vi "Init Trigger Output.vi"(8 "Error in":errorcluster, 11 "State Variables in":T1={"Stop Notifier"=refnum, "UI References"=[], "DAQmx"={"ECG Input"={"Channel"="", "Task"="", "Max Value"=0.0, "Min Value"=0.0, "Sampling Rate"=0.0, "Batch Size"=10}, "Trigger Output"={"Channel"="", "Task"="", "Pulse Frequency"=0.0, "Delay"=0, "Triggers per Shot"=0}}, "Data Queue"=refnum, "Filter"={"Batch Size"=1000, "Update Cycle"=0, "Filter Buffer"=[]}, "Last Detect Result"=FALSE}) -> (0 "Error out":errorcluster, 3 "State Variables out":T1={"Stop Notifier"=refnum, "UI References"=[], "DAQmx"={"ECG Input"={"Channel"="", "Task"="", "Max Value"=0.0, "Min Value"=0.0, "Sampling Rate"=0.0, "Batch Size"=10}, "Trigger Output"={"Channel"="", "Task"="", "Pulse Frequency"=0.0, "Delay"=0, "Triggers per Shot"=0}}, "Data Queue"=refnum, "Filter"={"Batch Size"=1000, "Update Cycle"=0, "Filter Buffer"=[]}, "Last Detect Result"=FALSE})   [LabVIEW 2014, in "Trigger Output.lvlib"]
uses:
  Trigger Output.lvlib
  Controls/State Variables.ctl
  Controls/DAQmx Variables.ctl
  Controls/Filter Variables.ctl
  <vilib>/DAQmx/create/channels.llb/DAQmx Create Channel (CO-Pulse Generation-Frequency).vi
  <vilib>/DAQmx/configure/timing.llb/DAQmx Timing (Implicit).vi
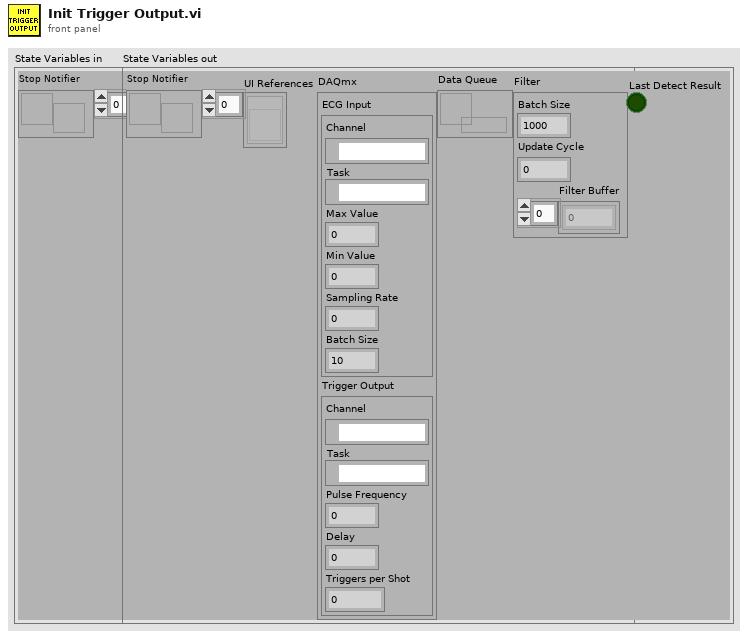
[diagram p1: front panel]
types:
  T1 = typedef "State Variables.ctl" = cluster{"Stop Notifier":refnum<notifier>, "UI References":refnum<vi>[], "DAQmx":T2, "Data Queue":refnum<queue>, "Filter":T3, "Last Detect Result":bool}
  T2 = typedef "DAQmx Variables.ctl" = cluster{"ECG Input":cluster{"Channel":tag, "Task":refnum<k21>, "Max Value":dbl, "Min Value":dbl, "Sampling Rate":dbl, "Batch Size":i32}, "Trigger Output":cluster{"Channel":tag, "Task":refnum<k21>, "Pulse Frequency":dbl, "Delay":u16, "Triggers per Shot":i32}}
  T3 = typedef "Filter Variables.ctl" = cluster{"Batch Size":i32, "Update Cycle":i32, "Filter Buffer":dbl[]}
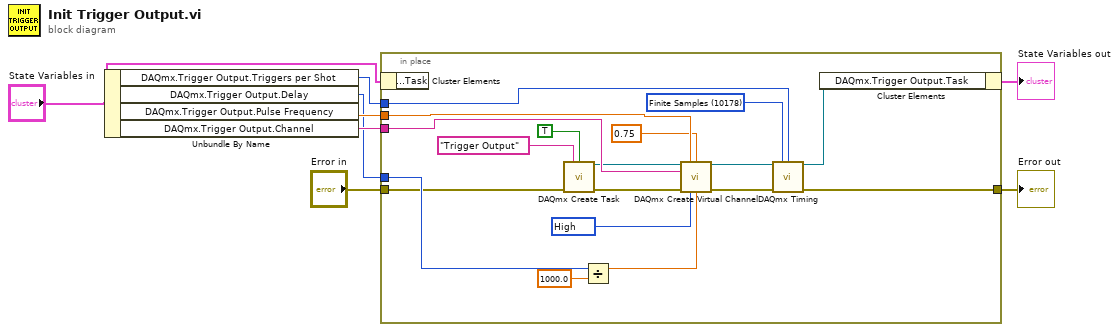
[diagram p0: block diagram]
diagram:
  n1 = Unbundle By Name("State Variables in") -> ("DAQmx.Trigger Output.Triggers per Shot"=w1:i32, "DAQmx.Trigger Output.Delay"=w2:u16, "DAQmx.Trigger Output.Pulse Frequency"=w3:dbl, "DAQmx.Trigger Output.Channel"=w6:tag)
  n2 = in-place {
    in-place-border: w6 -> [w24]
    in-place-border: "Error in" -> [w14]
    in-place-border: [w23] -> w4
    in-place-border: w3 -> [w21]
    in-place-border: w2 -> [w20]
    in-place-border: w1 -> [w17]
    w16 = 10178 items=["Finite Samples"=10178, "Continuous Samples"=10123, "Hardware Timed Single Point"=12522] ("sample mode")
    w19 = 10192 items=["High"=10192, "Low"=10214] ("idle state")
    n3 = in-place-cluster #1("State Variables in") -> ()  [unwired: 1 out]
    n4 = call <vilib>:"DAQmx Create Task.vi"("new task name"="Trigger Output" ("name to assign"), "auto cleanup"=TRUE, "error in"=w14) -> ("task out"=w12:refnum<k21>, "error out"=w13:errorcluster)  [unwired: 11 in]
    n5 = Divide(x=w20, y=1000.0) -> (x/y=w10:dbl)
    n6 = call-poly <vilib>:"DAQmx Create Virtual Channel.vi"("task in"=w12, "frequency"=w21, "duty cycle"=0.75, "counter"=w24, "error in"=w13, "idle state"=w19, "initial delay"=w10) -> ("task out"=w26:refnum<k21>, "error out"=w25:errorcluster)  [unwired: 7 in]
    n7 = call-poly <vilib>:"DAQmx Timing.vi"("task/channels in"=w26, "sample mode"=w16, "samples per channel"=w17, "error in"=w25) -> ("task out"=w22:refnum<k21>, "error out"=w23:errorcluster)  [unwired: 10 in]
    n8 = in-place-cluster #1("DAQmx.Trigger Output.Task"=w22) -> (→"State Variables out":T1)
  }
  "Error out" <- w4
